vi "告警码字段定义.vi"(7 "id":u16, 11 "告警代码":u16) -> (3 "告警信息":T1)   [LabVIEW 2016, in "斯坦道氨氮.lvlib"]
uses:
  Alarm interface/Alarm interface.lvlib
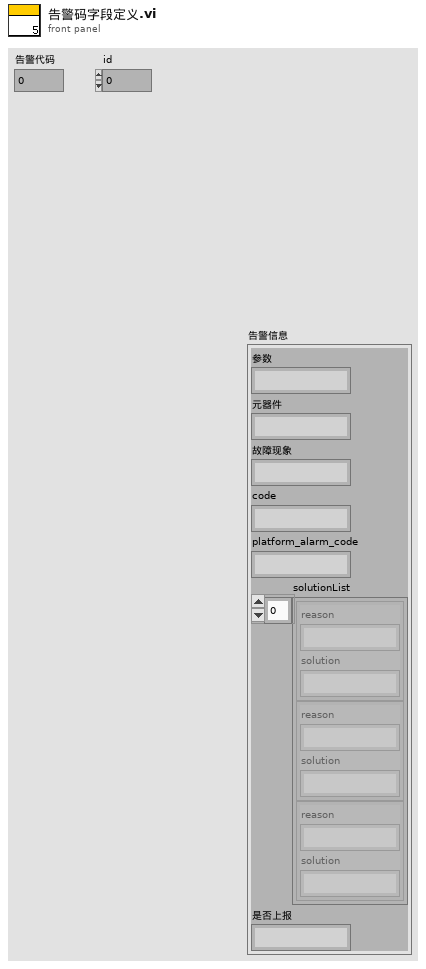
[diagram p1: front panel]
types:
  T1 = typedef "Alarm interface.lvlib/报警短信语音交互.ctl" = cluster{"参数":string, "元器件":string, "故障现象":string, "code":string, "platform_alarm_code":string, "solutionList":cluster{"reason":string, "solution":string}[], "是否上报":string}
  T2 = typedef "Alarm interface.lvlib/map in.ctl" = cluster{"name":string, "CN":string, "FirmwareVersion":string, "code":string}
  T3 = typedef "SingleStepTestV3.lvlib/SingleStepTestV3.lvclass/仪器版本.ctl" = enum16{"V3.1版", "V4版", "V3版", "V4.2版"}
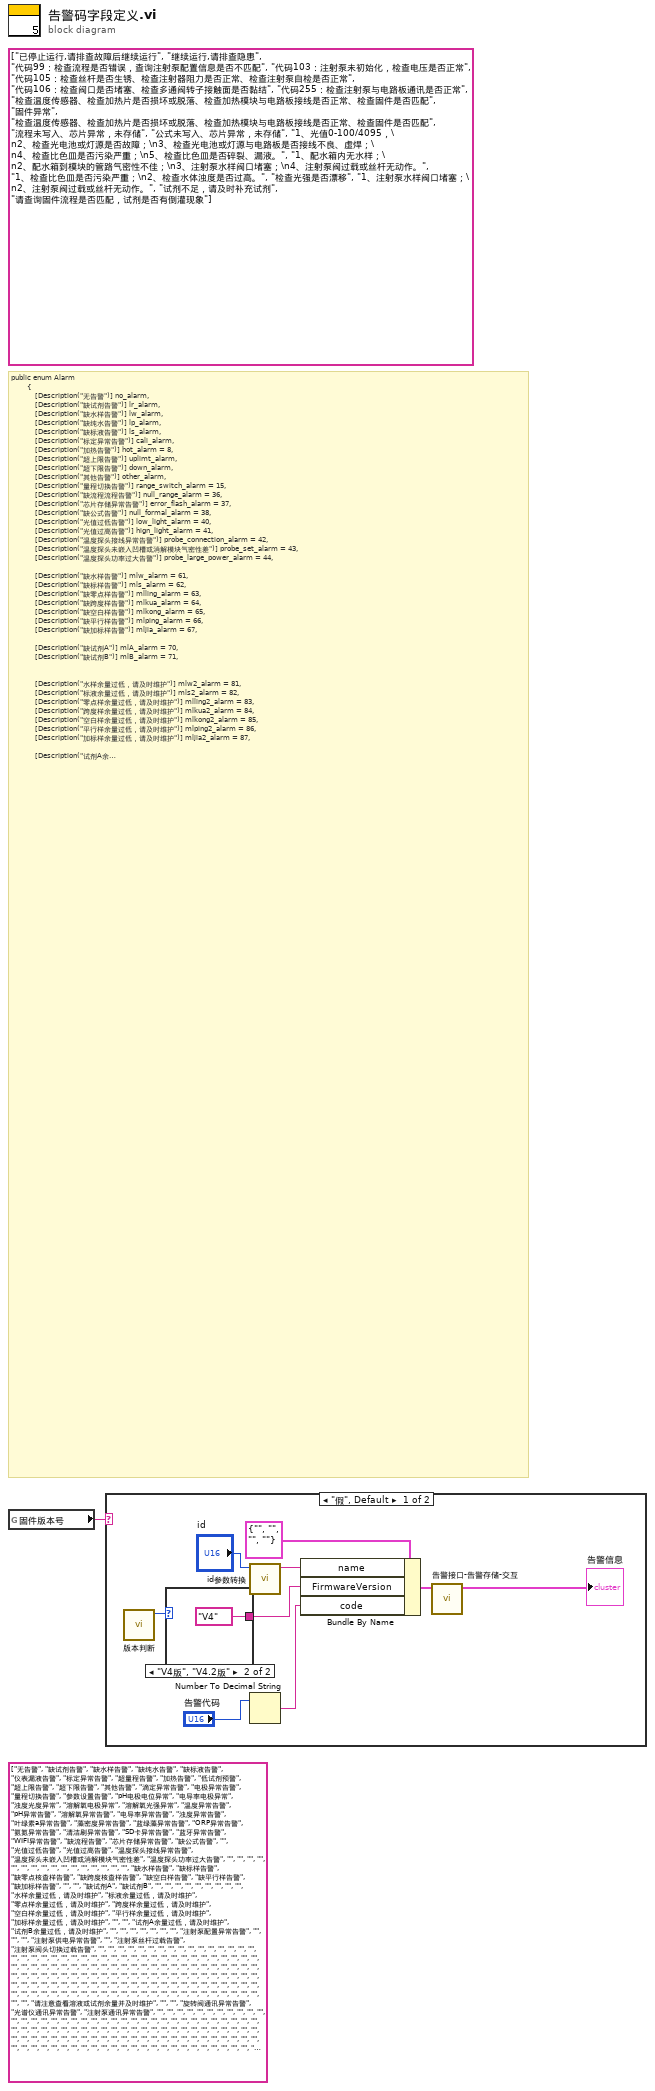
[diagram p0: block diagram]
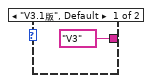
[diagram p2: hidden frame]
diagram:
  (unwired) string[] ["无告警", "缺试剂告警", "缺水样告警", "缺纯水告警", "缺标液告警", "仪表漏液告警", "标定异常告警", "超量程告警", "加热告警", "低试剂预警", "超上限告警", "超下限告警", "其他告警", "滴定异常告警", "电极异常告警", "量程切换告警", "参数设置告警", "pH电极电位异常", "电导率电极异常", "浊度光度异常", "溶解氧电极异常", "溶解氧光强异常", "温度异常告警", "pH异常告警", "溶解氧异常告警", "电导率异常告警", "浊度异常告警", "叶绿素a异常告警", "藻密度异常告警", "蓝绿藻异常告警", "ORP异常告警", "氨氮异常告警", "清洁刷异常告警", "SD卡异常告警", "蓝牙异常告警", "WIFI异常告警", "缺流程告警", "芯片存储异常告警", "缺公式告警", "", "光值过低告警", "光值过高告警", "温度探头接线异常告警", "温度探头未嵌入凹槽或消解模块气密性差", "温度探头功率过大告警", "", "", "", "", "", "", "", "", "", "", "", "", "", "", "", "", "缺水样告警", "缺标样告警", "缺零点核查样告警", "缺跨度核查样告警", "缺空白样告警", "缺平行样告警", "缺加标样告警", "", "", "缺试剂A", "缺试剂B", "", "", "", "", "", "", "", "", "", "水样余量过低，请及时维护", "标液余量过低，请及时维护", "零点样余量过低，请及时维护", "跨度样余量过低，请及时维护", "空白样余量过低，请及时维护", "平行样余量过低，请及时维护", "加标样余量过低，请及时维护", "", "", "试剂A余量过低，请及时维护", "试剂B余量过低，请及时维护", "", "", "", "", "", "", "", "注射泵配置异常告警", "", "", "", "注射泵供电异常告警", "", "注射泵丝杆过载告警", "注射泵阀头切换过载告警", "", "", "", "", "", "", "", "", "", "", "", "", "", "", "", "", "", "", "", "", "", "", "", "", "", "", "", "", "", "", "", "", "", "", "", "", "", "", "", "", "", "", "", "", "", "", "", "", "", "", "", "", "", "", "", "", "", "", "", "", "", "", "", "", "", "", "", "", "", "", "", "", "", "", "", "", "", "", "", "", "", "", "", "", "", "", "", "", "", "", "", "", "", "", "", "", "", "", "", "", "", "", "", "", "", "", "", "", "", "", "", "", "", "", "", "", "", "", "", "", "", "", "", "", "", "", "", "", "", "", "", "", "", "", "", "", "", "", "", "", "", "", "", "请注意查看溶液或试剂余量并及时维护", "", "", "旋转阀通讯异常告警", "光谱仪通讯异常告警", "注射泵通讯异常告警", "", "", "", "", "", "", "", "", "", "", "", "", "", "", "", "", "", "", "", "", "", "", "", "", "", "", "", "", "", "", "", "", "", "", "", "", "", "", "", "", "", "", "", "", "", "", "", "", "", "", "", "", "", "", "", "", "", "", "", "", "", "", "", "", "", "", "", "", "", "", "", "", "", "", "", "", "", "", "", "", "", "", "", "", "", "", "", "", "", "", "", "", "", "", "", "", "", "", "", "", "", "", "", "", "", "", "", "", "", "", "", "", "", "", "", "", "", "", "", "", "", "", "", "", "", "", "", "", "", "", "", "", "", "", "", "", "", "", "", "", "", "", "", "", "", "", "", "", "", "", "", "", "", "", "", "", "", "", "", "", "", "", "", "", "", "", "", "", "", "", "", "", "", "", "", "", "", "", "", "", "", "", "", "", "", "", "", "", "", "", "", "", "", "", "", "", "", "", "", "", "", "", "", "", "", "", "", "", "", "", "", "", "", "", "", "", "", "", "", "", "", "", "", "", "", "", "", "", "", "", "", "", "", "", "", "", "", "", "", "", "", "", "", "", "试剂不足", "试剂余量检测异常"]
  (unwired) string[] ["已停止运行,请排查故障后继续运行", "继续运行,请排查隐患", "代码99：检查流程是否错误，查询注射泵配置信息是否不匹配", "代码103：注射泵未初始化，检查电压是否正常", "代码105：检查丝杆是否生锈、检查注射器阻力是否正常、检查注射泵自检是否正常", "代码106：检查阀口是否堵塞、检查多通阀转子接触面是否黏结", "代码255：检查注射泵与电路板通讯是否正常", "检查温度传感器、检查加热片是否损坏或脱落、检查加热模块与电路板接线是否正常、检查固件是否匹配", "固件异常", "检查温度传感器、检查加热片是否损坏或脱落、检查加热模块与电路板接线是否正常、检查固件是否匹配", "流程未写入、芯片异常，未存储", "公式未写入、芯片异常，未存储", "1、光值0-100/4095，\n2、检查光电池或灯源是否故障；\n3、检查光电池或灯源与电路板是否接线不良、虚焊；\n4、检查比色皿是否污染严重；\n5、检查比色皿是否碎裂、漏液。", "1、配水箱内无水样；\n2、配水箱到模块的管路气密性不佳；\n3、注射泵水样阀口堵塞；\n4、注射泵阀过载或丝杆无动作。", "1、检查比色皿是否污染严重；\n2、检查水体浊度是否过高。", "检查光强是否漂移", "1、注射泵水样阀口堵塞；\n2、注射泵阀过载或丝杆无动作。", "试剂不足，请及时补充试剂", "请查询固件流程是否匹配，试剂是否有倒灌现象"]
  # "public enum Alarm\n        {\n            [Description(\"无告警\")] no_alarm,\n            [Description(\"缺试剂告警\")] lr_alarm,\n            [Description(\"缺水样告警\")] lw_alarm,\n            [Description(\"缺纯水告警\")] lp_alarm,\n            [Description(\"缺标液告警\")] ls_alarm,\n            [Description(\"标定异常告警\")] cali_alarm,\n            [Description(\"加热告警\")] hot_alarm = 8,\n            [Description(\"超上限告警\")] uplimt_alarm,\n            [Description(\"超下限告警\")] down_alarm,\n            [Description(\"其他告警\")] other_alarm,\n            [Description(\"量程切换告警\")] range_switch_alarm = 15,\n            [Description(\"缺流程流程告警\")] null_range_alarm = 36,\n            [Description(\"芯片存储异常告警\")] error_flash_alarm = 37,\n            [Description(\"缺公式告警\")] null_formal_alarm = 38,\n            [Description(\"光值过低告警\")] low_light_alarm = 40,\n            [Description(\"光值过高告警\")] hign_light_alarm = 41,\n            [Description(\"温度探头接线异常告警\")] probe_connection_alarm = 42,\n            [Description(\"温度探头未嵌入凹槽或消解模块气密性差\")] probe_set_alarm = 43,\n            [Description(\"温度探头功率过大告警\")] probe_large_power_alarm = 44,\n\n            [Description(\"缺水样告警\")] mlw_alarm = 61,\n            [Description(\"缺标样告警\")] mls_alarm = 62,\n            [Description(\"缺零点样告警\")] mlling_alarm = 63,\n            [Description(\"缺跨度样告警\")] mlkua_alarm = 64,\n            [Description(\"缺空白样告警\")] mlkong_alarm = 65,\n            [Description(\"缺平行样告警\")] mlping_alarm = 66,\n            [Description(\"缺加标样告警\")] mljia_alarm = 67,\n\n            [Description(\"缺试剂A\")] mlA_alarm = 70,\n            [Description(\"缺试剂B\")] mlB_alarm = 71,\n\n\n            [Description(\"水样余量过低，请及时维护\")] mlw2_alarm = 81,\n            [Description(\"标液余量过低，请及时维护\")] mls2_alarm = 82,\n            [Description(\"零点样余量过低，请及时维护\")] mlling2_alarm = 83,\n            [Description(\"跨度样余量过低，请及时维护\")] mlkua2_alarm = 84,\n            [Description(\"空白样余量过低，请及时维护\")] mlkong2_alarm = 85,\n            [Description(\"平行样余量过低，请及时维护\")] mlping2_alarm = 86,\n            [Description(\"加标样余量过低，请及时维护\")] mljia2_alarm = 87,\n\n            [Description(\"试剂A余量过低，请及时维护\")] mlA2_alarm = 90,\n            [Description(\"试剂B余量过低，请及时维护\")] mlB2_alarm = 91,\n\n\n            [Description(\"注射泵供电告警\")] pump_Not_Initialized_alarm = 103,\n            [Description(\"注释泵丝杆过载过载告警\")] pump_Plunger_Overload_alarm = 105,\n            [Description(\"注释泵阀头切换过载告警\")] pump_Valve_Overload_alarm = 106,\n            [Description(\"注射泵配置异常告警\")] pump_Valve_Config_alarm = 99,\n            [Description(\"请注意查看溶液或试剂余量并及时维护\")] reagentRemaid_alarm = 250,\n            [Description(\"旋转阀通信异常告警\")] valve_commuication_alarm = 253,\n            [Description(\"光谱仪通信异常告警\")] spec_commuication_alarm = 254,\n            [Description(\"注射泵通信异常告警\")] pump_commuication_alarm = 255,\n        }\n        public enum Error\n        {\n            [Description(\"无故障\")] no_error,\n            [Description(\"注射泵故障\")] pump_error,\n            [Description(\"加热故障\")] hot_error,\n            [Description(\"旋转阀故障\")] value_error,\n\n            [Description(\"光值过低故障\")] low_light_error = 38,\n            [Description(\"光路系统故障\")] error_light_error = 39,\n        }"
  n1 = global read "VAR总磷总氮全局变量.vi" "固件版本号"() -> (w1:string)
  n2 = case shown="\"假\", Default" w1 {
    frame "假", Default {
      n3 = call "版本判断.vi"() -> ("仪器版本"=w5:T3)  [unwired: 11 in]
      n4 = case shown="\"V4版\", \"V4.2版\"" w5 {
        tunnel: ["V3" ("equipVersion") "V4" ("equipVersion")] -> w4
        frame "V3.1版", Default {
        }
        frame "V4版", "V4.2版" {
        }
      }
      n5 = call "id参数转换.vi"("id"="id") -> ("table输出"=w6:string)  [unwired: 9 in, 1 out]
      n6 = Number To Decimal String(number="告警代码") -> (decimal integer string=w8:string)  [unwired: 1 in]
      n7 = Bundle By Name(cluster=T2 {"name"="", "CN"="", "FirmwareVersion"="", "code"=""} ("map in"), "name"=w6, "FirmwareVersion"=w4, "code"=w8) -> (w2:T2)
      n8 = call "告警接口-告警存储-交互.vi"("map in"=w2) -> ("data"=→"告警信息":T1)  [unwired: 10 in]
    }
    frame "" {
    }
  }
